vi "Distance rayon a faisceau.vi"(9 "T ambiant":dbl, 10 "T max":dbl, 11 "T capteur":dbl) -> (3 "Rayon":dbl)   [LabVIEW 2018]
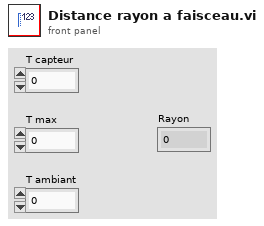
[diagram p1: front panel]
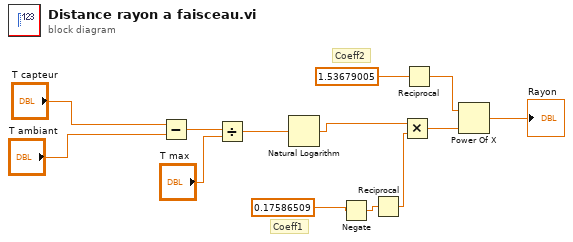
[diagram p0: block diagram]
diagram:
  # "Coeff2"
  # "Coeff1"
  n1 = Subtract(x="T capteur", y="T ambiant") -> (x-y=w11:dbl)
  n2 = Divide(x=w11, y="T max") -> (x/y=w9:dbl)
  n3 = Natural Logarithm(1:w9) -> (0:w8:dbl)
  n4 = Negate(x=0.17586509) -> (-x=w6:dbl)
  n5 = Reciprocal(x=w6) -> (1/x=w7:dbl)
  n6 = Multiply(x=w8, y=w7) -> (x*y=w3:dbl)
  n7 = Reciprocal(x=1.53679005) -> (1/x=w2:dbl)
  n8 = Power Of X(1:w3, 2:w2) -> (0:→"Rayon":dbl)
